vi "controlEotOutputDeactive.vi"(7 "Set":bool, 8 "error in":errorcluster, 9 "Enabled":bool, 10 "axis in":u8, 11 "connection ID":refnum<k5>) -> (0 "error out":errorcluster, 1 "Enabled out":bool, 2 "axis out":i32, 3 "connection ID":refnum<k5>)   [LabVIEW 2015, in "AMC_VIs.lvlib"]
doc: "This function retrieves or sets the output applied to the selected axis on the end of travel."
uses:
  AMC_VIs.lvlib
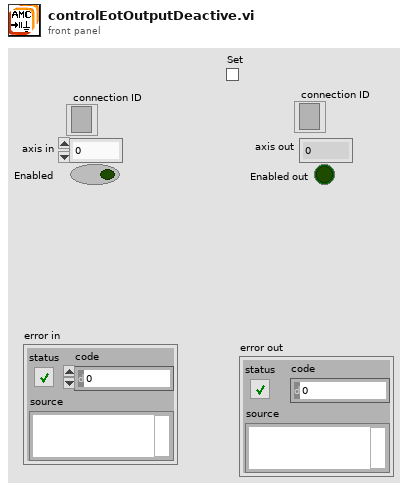
[diagram p1: front panel]
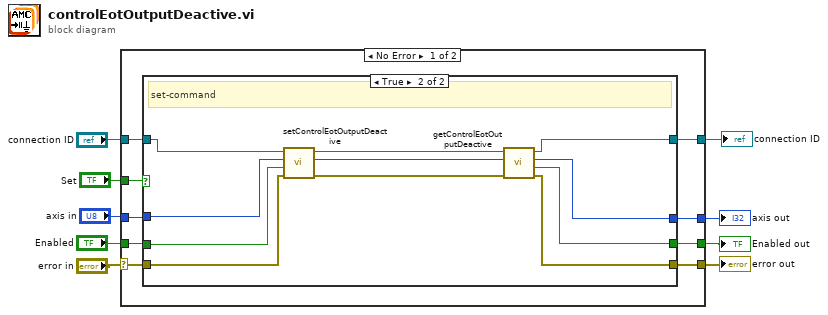
[diagram p0: block diagram]
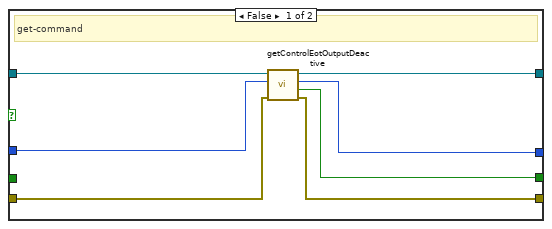
[diagram p2: hidden frame]
diagram:
  n1 = case shown="No Error" "error in" {
    selector: "error in" -> [w14 w40]
    tunnel: "axis in" -> [w18 w37]
    tunnel: [w12 w40] -> w8
    tunnel: "Enabled" -> [w16 w38]
    tunnel: [w13 w38] -> w3
    tunnel: "Set" -> [w15 _]
    tunnel: [w11 w39] -> w6
    tunnel: "connection ID" -> [w17 w39]
    tunnel: [w10 w37] -> w1
    frame No Error {
      n2 = case shown="True" w15 {
        tunnel: w17 -> [w20 w33]
        tunnel: w18 -> [w19 w29]
        tunnel: w16 -> [_ w28]
        tunnel: w14 -> [w25 w36]
        tunnel: [w23 w26] -> w13
        tunnel: [w24 w34] -> w12
        tunnel: [w21 w31] -> w11
        tunnel: [w22 w27] -> w10
        frame False {
          # "get-command"
          n3 = call "getControlEotOutputDeactive.vi"("error in"=w25, "axis"=w19, "connection ID"=w20) -> ("error out"=w24:errorcluster, "enabled"=w23:bool, "axis_out"=w22:i32, "connection ID"=w21:refnum<k5>)  [unwired: 5 in]
        }
        frame True {
          # "set-command"
          n4 = call "setControlEotOutputDeactive.vi"("error in"=w36, "enable"=w28, "axis"=w29, "connection ID"=w33) -> ("error out"=w35:errorcluster, "axis_out"=w30:i32, "connection ID"=w32:refnum<k5>)  [unwired: 5 in]
          n5 = call "getControlEotOutputDeactive.vi"("error in"=w35, "axis"=w30, "connection ID"=w32) -> ("error out"=w34:errorcluster, "enabled"=w26:bool, "axis_out"=w27:i32, "connection ID"=w31:refnum<k5>)  [unwired: 5 in]
        }
      }
    }
    frame Error {
    }
  }
  "error out" <- w8
  "axis out" <- w1
  "Enabled out" <- w3
  "connection ID" <- w6
